vi "XYStage.KIM101.GetPrivateEventsRegistration.vi"(8 "error in (no error)":errorcluster, 11 "XYStage.KIM101 in":refnum<class "XYStage.KIM101.lvclass">) -> (0 "error out":errorcluster, 2 "XYStage.KIM101 Private Events":refnum<event-registration>, 3 "XYStage.KIM101 out":refnum<class "XYStage.KIM101.lvclass">)   [LabVIEW 2017, in "XYStage.KIM101.lvclass"]
uses:
  XYStage.KIM101.lvclass
  Typedefs/PrivateEvents--Cluster.ctl
  Typedefs/PrivateEvents--XYStage.KIM101.MoveAbsolute (counts).ctl
  XYStage/Typedefs/Coordinates.Counts--Cluster.ctl
  XYStage/XYStage.lvclass
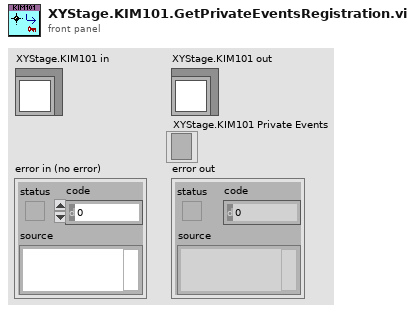
[diagram p1: front panel]
types:
  T1 = typedef "XYStage.KIM101.lvclass/PrivateEvents--Cluster.ctl" = cluster{"MoveAbsolute (counts)":refnum<user-event>}
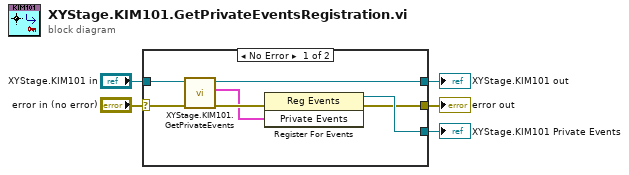
[diagram p0: block diagram]
diagram:
  n1 = case shown="No Error" "error in (no error)" {
    selector: "error in (no error)" -> [w9 w14]
    tunnel: [w6 w14] -> w4
    tunnel: [w8 w13] -> w2
    tunnel: "XYStage.KIM101 in" -> [w12 w13]
    tunnel: [w7 _] -> w1
    frame No Error {
      n2 = call "XYStage.KIM101.GetPrivateEvents.vi"("error in (no error)"=w9, "XYStage.KIM101 in"=w12) -> ("error out"=w11:errorcluster, "Private Events"=w10:T1, "XYStage.KIM101 out"=w8:refnum<class "XYStage.KIM101.lvclass">)  [unwired: 7 in]
      n3 = register-events(error in=w11, w10) -> (reference out=w7:refnum<event-registration>, error out=w6:errorcluster)  [unwired: 1 in]
    }
    frame Error {
    }
  }
  "error out" <- w4
  "XYStage.KIM101 out" <- w2
  "XYStage.KIM101 Private Events" <- w1
